vi "Search for Home.vi"(8 "error in (no error)":errorcluster, 10 "Axis":i32, 11 "Home Mode":T1) -> (0 "error out":errorcluster)   [LabVIEW 2019, in "ESP301.lvlib"]
doc: "_____\nCreated using Delacor QMH Event Scripter 5.0.0.112."
uses:
  ESP301.lvlib
  Home Mode.ctl
  Search for Home Argument--cluster.ctl
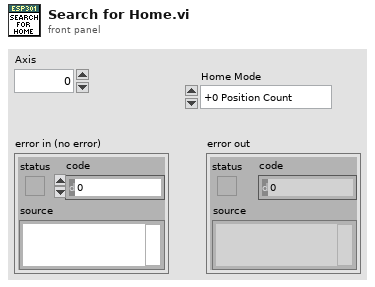
[diagram p1: front panel]
types:
  T1 = typedef "Home Mode.ctl" = enum16{"+0 Position Count", "Home and Index Singals", "Home Signal", "Positive Limit Signal", "Negative Limit Signal", "Positive Limit Signal and Index Signals", "Negative Limit Signal and Index Signals"}
  T2 = typedef "ESP301.lvlib/Search for Home Argument--cluster.ctl" = cluster{"Axis":i32, "Home Mode":T1}
  T3 = typedef "ESP301.lvlib/Request Events--cluster.ctl" = cluster{"Stop Module":refnum<user-event>, "Show Panel":refnum<user-event>, "Hide Panel":refnum<user-event>, "Get Module Execution Status":refnum<user-event>, "Show Diagram":refnum<user-event>, "Set Position":refnum<user-event>, "Get Position":refnum<user-event>, "Search for Home":refnum<user-event>}
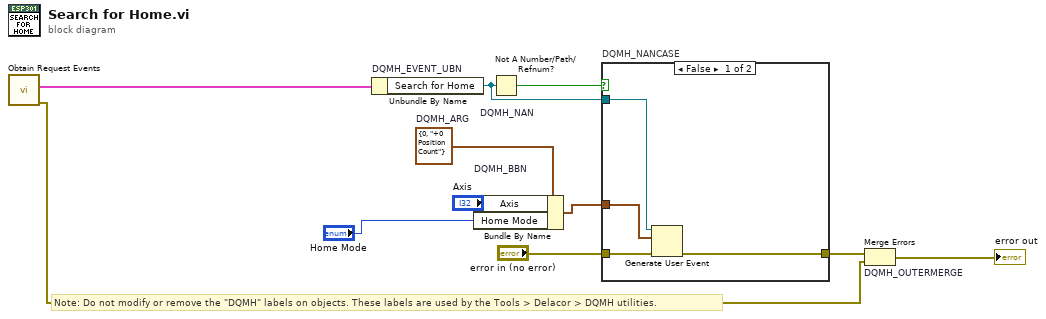
[diagram p0: block diagram]
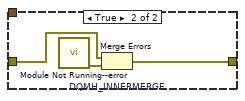
[diagram p2: hidden frame]
diagram:
  w5 = T2 {"Axis"=0, "Home Mode"=enum."+0 Position Count"}  # DQMH_ARG
  # "Note: Do not modify or remove the \"DQMH\" labels on objects. These labels are used by the Tools > Delacor > DQMH utilities."
  n1 = call "Obtain Request Events.vi"() -> ("error out"=w3:errorcluster, "ESP301 Request Events"=w2:T3)  [unwired: 10 in]
  n2 = Unbundle By Name "DQMH_EVENT_UBN"(w2) -> ("Search for Home"=w7:refnum<user-event>)
  n3 = Bundle By Name "DQMH_BBN"(cluster=w5, "Axis"="Axis", "Home Mode"="Home Mode") -> (w9:T2)
  n4 = Not A Number/Path/Refnum? "DQMH_NAN"(number/path/refnum=w7) -> (NaN/Path/Refnum?=w8:bool)
  n5 = case "DQMH_NANCASE" shown="False" w8 {
    tunnel: "error in (no error)" -> [w15 w18]
    tunnel: [w14 w17] -> w6
    tunnel: w7 -> [w13 _]
    tunnel: w9 -> [w12 _]
    frame False {
      n6 = Generate User Event(user event=w13, event data cluster=w12, error in=w15) -> (error out=w14:errorcluster)  [unwired: 1 in, 1 out]
    }
    frame True {
      n7 = call "Module Not Running--error.vi"() -> ("error out"=w16:errorcluster)  [unwired: 11 in]
      n8 = Merge Errors "DQMH_INNERMERGE"(w18, w16) -> (w17:errorcluster)
    }
  }
  n9 = Merge Errors "DQMH_OUTERMERGE"(w6, w3) -> (→"error out":errorcluster)
